vi "Measurement.vi"(8 "error in (no error)":errorcluster, 9 "timeout":u32, 10 "Meter ID":i32, 11 "FieldMax2Lib.dll path":path) -> (0 "error out":errorcluster, 1 "Measurement Value":sgl, 2 "Meter ID":i32, 3 "FieldMax2Lib.dll path":path)   [LabVIEW 2012]
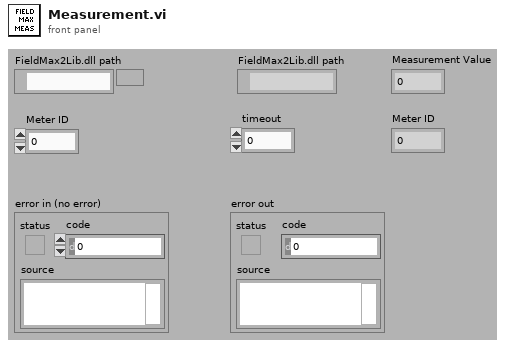
[diagram p1: front panel]
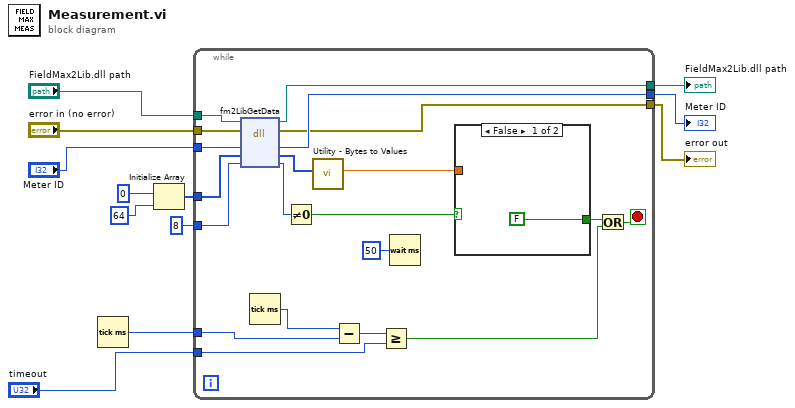
[diagram p0: block diagram]
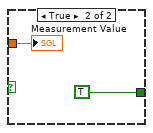
[diagram p2: hidden frame]
diagram:
  n1 = Tick Count (ms)() -> (millisecond timer value=w2:u32)
  n2 = Initialize Array(u8 0 ("element"), 64 ("dimension size")) -> (w10:u8[])
  n3 = while {
    tunnel: w10 -> [w29]
    tunnel: i16 8 ("count") -> [w28]
    tunnel: [w25] -> w5
    tunnel: [w24] -> w4
    tunnel: "FieldMax2Lib.dll path" -> [w23]
    tunnel: "error in (no error)" -> [w22]
    tunnel: "Meter ID" -> [w21]
    tunnel: [w20] -> w3
    tunnel: w2 -> [w18]
    tunnel: "timeout" -> [w16]
    stop <- w14 stop-if-true
    n4 = dll-call lib="C:/Windows/System32/FieldMax2Lib.dll" fn="fm2LibGetData" label="Get Data"(path in=w23, error in=w22, "h"=w21, "returnBuffer"=w29, "count"=w28) -> (path out=w24:path, error out=w20:errorcluster, "h"=w25:i32, "returnBuffer"=w26:u8[], "count"=w27:i16)  [unwired: 2 in]
    n5 = Tick Count (ms)() -> (millisecond timer value=w19:u32)
    n6 = Not Equal To 0?(x=w27) -> (x != 0?=w30:bool)
    n7 = call "Utility - Bytes to Values.vi"("DataBuffer"=w26) -> ("Measurement Value"=w31:sgl)  [unwired: 9 in, 1 out]
    n8 = Subtract(x=w19, y=w18) -> (x-y=w17:u32)
    n9 = Greater Or Equal?(x=w17, y=w16) -> (x >= y?=w13:bool)
    n10 = Wait (ms)(milliseconds to wait=u32 50) -> ()  [unwired: 1 out]
    n11 = case shown="False" w30 {
      tunnel: w31 -> [_ w34]
      tunnel: [FALSE TRUE] -> w15
      frame False {
      }
      frame True {
        "Measurement Value" <- w34
      }
    }
    n12 = Or(x=w15, y=w13) -> (x .or. y?=w14:bool)
  }
  "Meter ID" <- w5
  "FieldMax2Lib.dll path" <- w4
  "error out" <- w3
